vi "Read-Reg.vi"(8 "error in (no error)":errorcluster, 11 "Modbus-Instr in":refnum<class "Modbus-Instr.lvclass">) -> (0 "error out":errorcluster, 2 "Modbus-Reg":u16[](array[numeric]), 3 "Modbus-Instr out":refnum<class "Modbus-Instr.lvclass">)   [LabVIEW 2021, in "Modbus-Instr.lvclass"]
uses:
  Modbus-Instr.lvclass
  Modbus-Instr.lvclass/Modbus-Instr.ctl
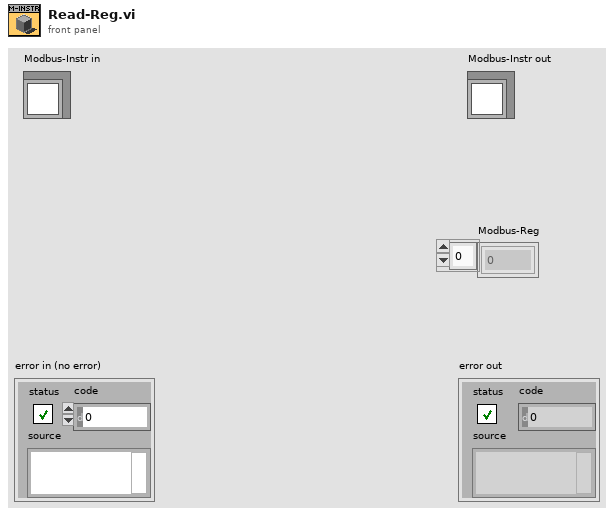
[diagram p1: front panel]
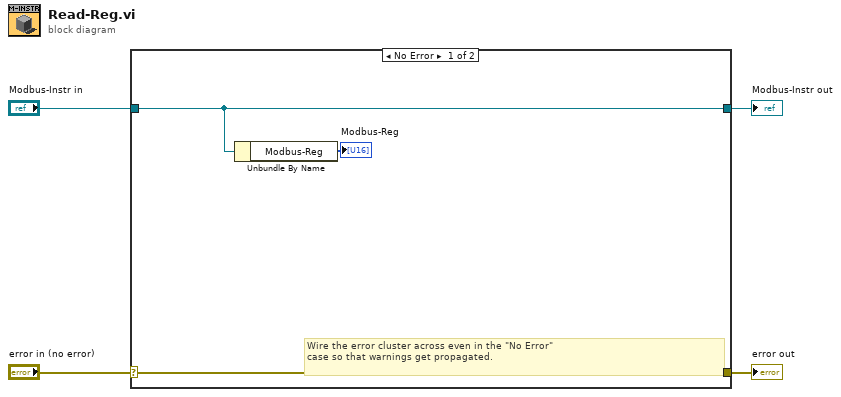
[diagram p0: block diagram]
diagram:
  n1 = case shown="No Error" "error in (no error)" {
    selector: "error in (no error)" -> [w7 w9]
    tunnel: [w7 w9] -> w3
    tunnel: [w6 w8] -> w1
    tunnel: "Modbus-Instr in" -> [w6 w8]
    frame No Error {
      # "Wire the error cluster across even in the \"No Error\"\ncase so that warnings get propagated."
      n2 = Unbundle By Name(w6) -> ("Modbus-Reg"=→"Modbus-Reg":u16[])
    }
    frame Error {
    }
  }
  "error out" <- w3
  "Modbus-Instr out" <- w1
